vi "Shutdown Sensor.vi"(8 "error in (no error)":errorcluster, 11 "Sensor in":refnum<class "Sensor.lvclass">) -> (0 "error out":errorcluster, 3 "Sensor out":refnum<class "Sensor.lvclass">)   [LabVIEW 2012, in "Sensor Definition.lvlib" / "Sensor.lvclass"]
uses:
  Sensor.lvclass
  Sensor.lvclass/Sensor.ctl
  <vilib>/ActorFramework/Message Enqueuer/Message Enqueuer.lvclass/Message Enqueuer.ctl
  <vilib>/ActorFramework/Actor/Actor.lvclass/Actor.ctl
  Read Listening SensorViews.vi
  <vilib>/ActorFramework/Message Enqueuer/Enqueue.vi
  <vilib>/ActorFramework/Message Enqueuer/Init from Existing Queue.vi
  <vilib>/ActorFramework/Message Priority Queue/Priority Enqueue.vi
  <vilib>/ActorFramework/Message Enqueuer/Message Enqueuer.lvclass
  <vilib>/ActorFramework/Stop Msg/Stop Msg.lvclass
  <vilib>/ActorFramework/Actor/Actor.lvclass
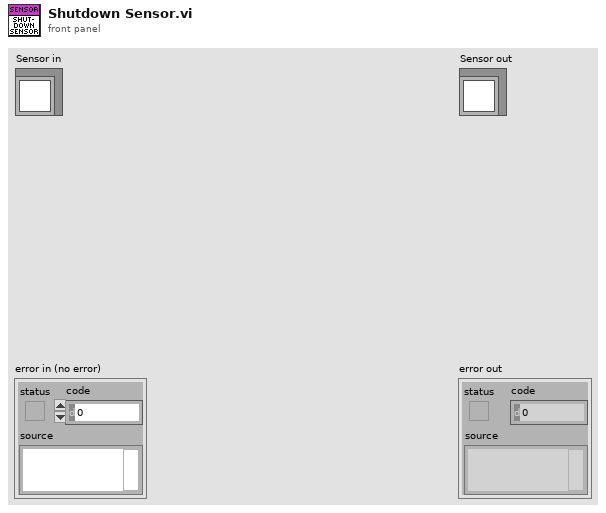
[diagram p1: front panel]
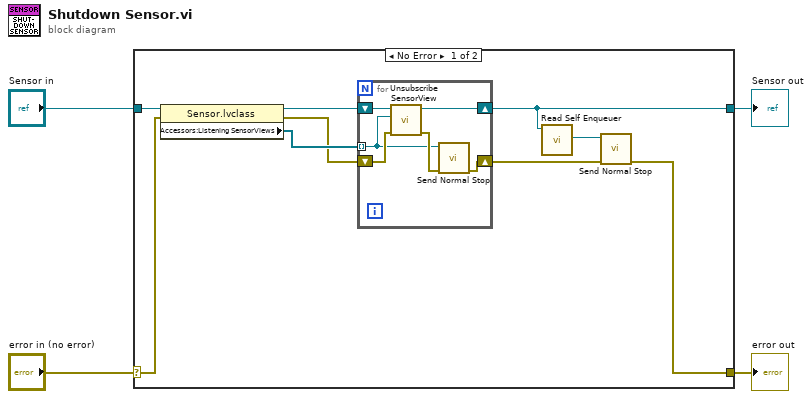
[diagram p0: block diagram]
diagram:
  n1 = case shown="No Error" "error in (no error)" {
    selector: "error in (no error)" -> [w6 w21]
    tunnel: [w5 w21] -> w3
    tunnel: [w10 w20] -> w1
    tunnel: "Sensor in" -> [w13 w20]
    frame No Error {
      n2 = property class="Sensor.lvclass"(reference=w13, error in=w6) -> (reference out=w12:refnum<class "Sensor.lvclass">, error out=w8:errorcluster, "Accessors:Listening SensorViews"=w11:refnum<class "Message Enqueuer.lvclass">[])
      n3 = for {
        shift-right: [w18] -> w10
        shift-left: w12 -> [w19]
        tunnel: w11 -> [w15] mode=indexing
        shift-right: [w14] -> w7
        shift-left: w8 -> [w17]
        n4 = call "Unsubscribe SensorView.vi"("error in (no error)"=w17, "SensorView Enqueuer"=w15, "Sensor in"=w19) -> ("error out"=w16:errorcluster, "Sensor out"=w18:refnum<class "Sensor.lvclass">)  [unwired: 7 in]
        n5 = call <vilib>:"Send Normal Stop.vi"("error in (no error)"=w16, "Message Enqueuer"=w15) -> ("error out"=w14:errorcluster)  [unwired: 9 in]
      }
      n6 = call <vilib>:"Read Self Enqueuer.vi"("Actor"=w10) -> ("Self Enqueuer"=w9:refnum<class "Message Enqueuer.lvclass">)  [unwired: 10 in]
      n7 = call <vilib>:"Send Normal Stop.vi"("error in (no error)"=w7, "Message Enqueuer"=w9) -> ("error out"=w5:errorcluster)  [unwired: 9 in]
    }
    frame Error {
    }
  }
  "error out" <- w3
  "Sensor out" <- w1
